vi "Execute_All_Process.vi"(6 "OperatorImage In":T1, 7 "MaskParam 2":refnum<vi>, 8 "error in (no error)":errorcluster, 9 "ImageIn":T1, 10 "ExtractImageIn":T1, 11 "ProcessSettingIn":T2[](array[typedef])) -> (0 "error out":errorcluster, 1 "Image Out":T1, 2 "ExtractImageOut":T1, 3 "Palette Type":u32, 4 "OperatorImage Out":T1, 5 "MaskParam 3":refnum<vi>)   [LabVIEW 2019]
uses:
  <vilib>/vision/Image Controls.llb/IMAQ Image.ctl
  Controls/Process_Setting.ctl
  Ctrl/VisionProcessName.ctl
panel:
  out "ProcessSettingOut":T2={"Enum_PreProcess"=enum."CamAttributes", "Parameter"=""}
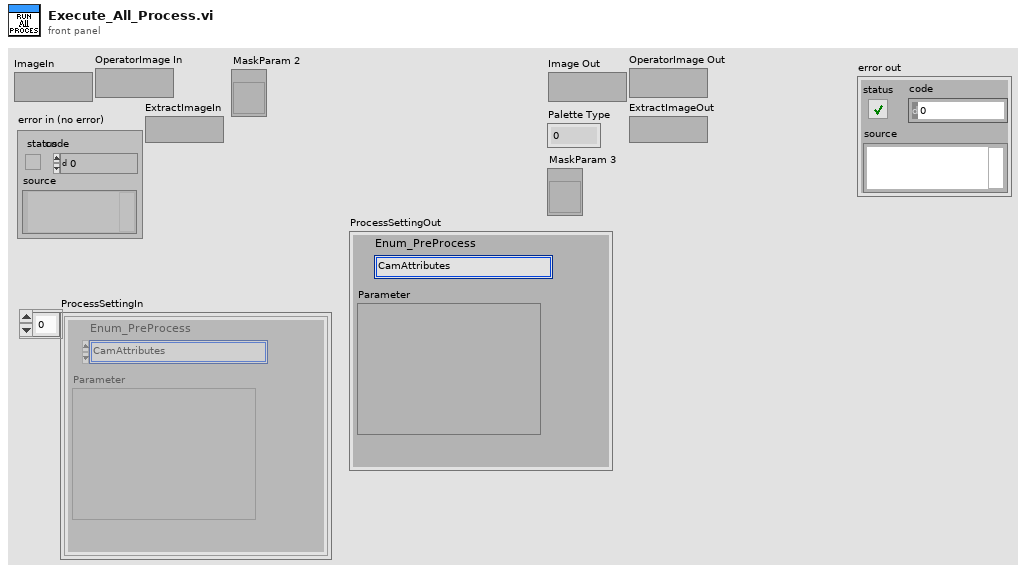
[diagram p1: front panel]
types:
  T1 = typedef "IMAQ Image.ctl" = refnum<image>
  T2 = typedef "Process_Setting.ctl" = cluster{"Enum_PreProcess":T3, "Parameter":string}
  T3 = typedef "VisionProcessName.ctl" = enum16{"*CamParameter*", "CamAttributes", "*Preprocess*", "CG_Brightness", "C_Plane Extraction", "C_Threshold", "G_Lookup Table", "G_Threshold"}
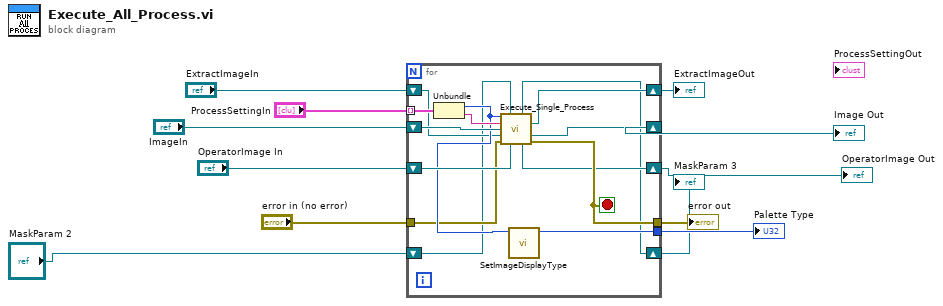
[diagram p0: block diagram]
diagram:
  n1 = for {
    tunnel: "ProcessSettingIn" -> [w24] mode=indexing
    shift-right: [w25] -> w10
    shift-left: "ImageIn" -> [w26]
    tunnel: [w20] -> w9
    shift-right: [w17] -> w5
    shift-left: "OperatorImage In" -> [w22]
    tunnel: "error in (no error)" -> [w19]
    tunnel: [w18] -> w6
    shift-right: [w16] -> w4
    shift-left: "ExtractImageIn" -> [w15]
    shift-right: [w13] -> w1
    shift-left: "MaskParam 2" -> [w14]
    stop <- w18 stop-if-true
    n2 = Unbundle(w24) -> ("Enum_PreProcess"=w21:T3, "Parameter"=w23:string)
    n3 = call "Execute_Single_Process.vi"("Tab Control"=w21, "MaskParam 2"=w14, "Parameter"=w23, "ImageIn"=w26, "ExtractImageControl"=w15, "error in (no error)"=w19, "OperatorImage"=w22) -> ("MaskParam 4"=w13:refnum<vi>, "ExtractImage"=w16:T1, "Image Out"=w25:T1, "OperatorImageOut"=w17:T1, "error out"=w18:errorcluster)  [unwired: 3 in, 1 out]
    n4 = call "SetImageDisplayType.vi"("Value"=w21) -> ("Palette:Palette Type"=w20:u32)  [unwired: 9 in, 1 out]
  }
  "error out" <- w6
  "Image Out" <- w10
  "Palette Type" <- w9
  "OperatorImage Out" <- w5
  "ExtractImageOut" <- w4
  "MaskParam 3" <- w1
